vi "DVL convert (SubVI).vi"(0 "String":string) -> (1 "depth":dbl, 3 "dvl alts":dbl[](array[numeric]), 4 "u_wt_dvl":dbl[](array[numeric]), 5 "u_bt_dvl":dbl[](array[numeric]), 6 "SA":dbl[](array[numeric]))   [LabVIEW 2014]
uses:
  Helping Routines/get_set_point (SubVI).vi
panel:
  in  "Reset pressure":bool
  out "BI":dbl[](array[numeric])
  out "WI":dbl[](array[numeric])
  out "RA":dbl[](array[numeric])
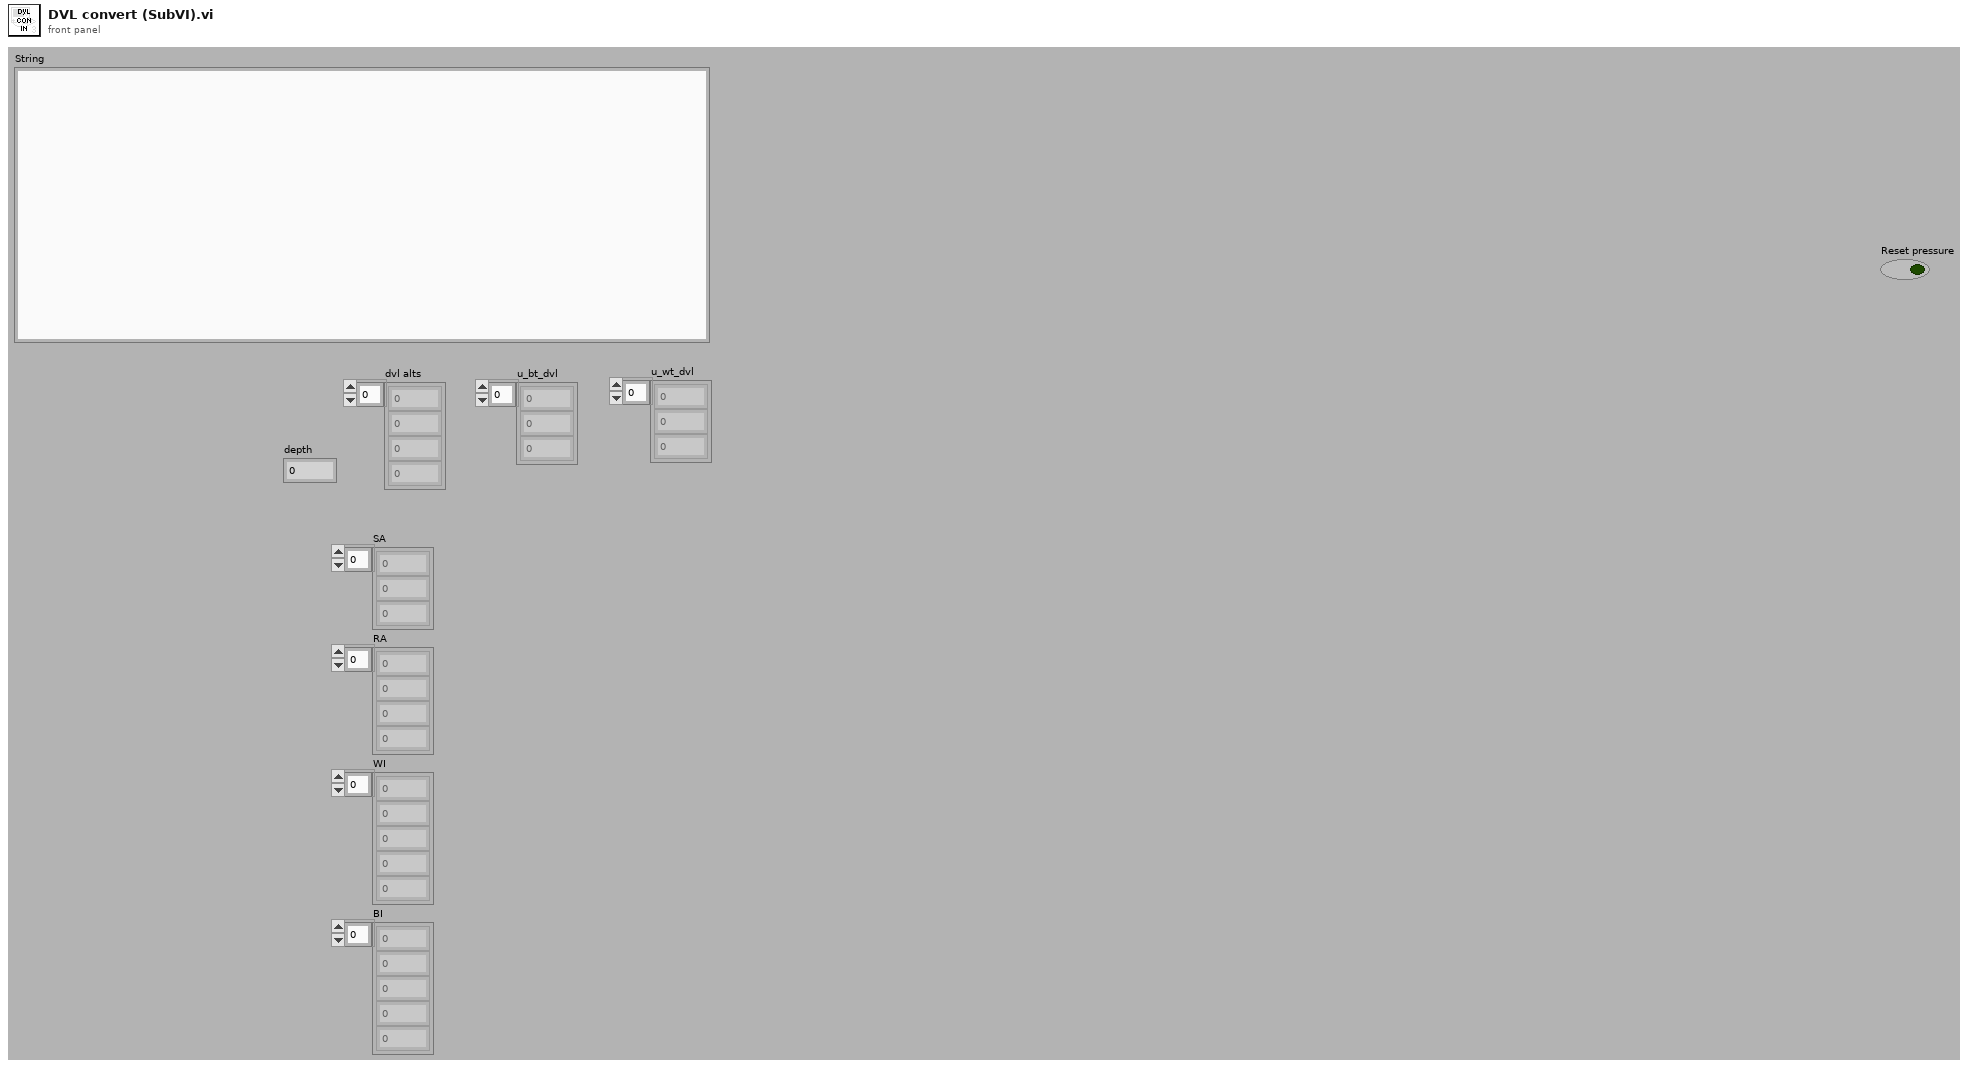
[diagram p1: front panel]
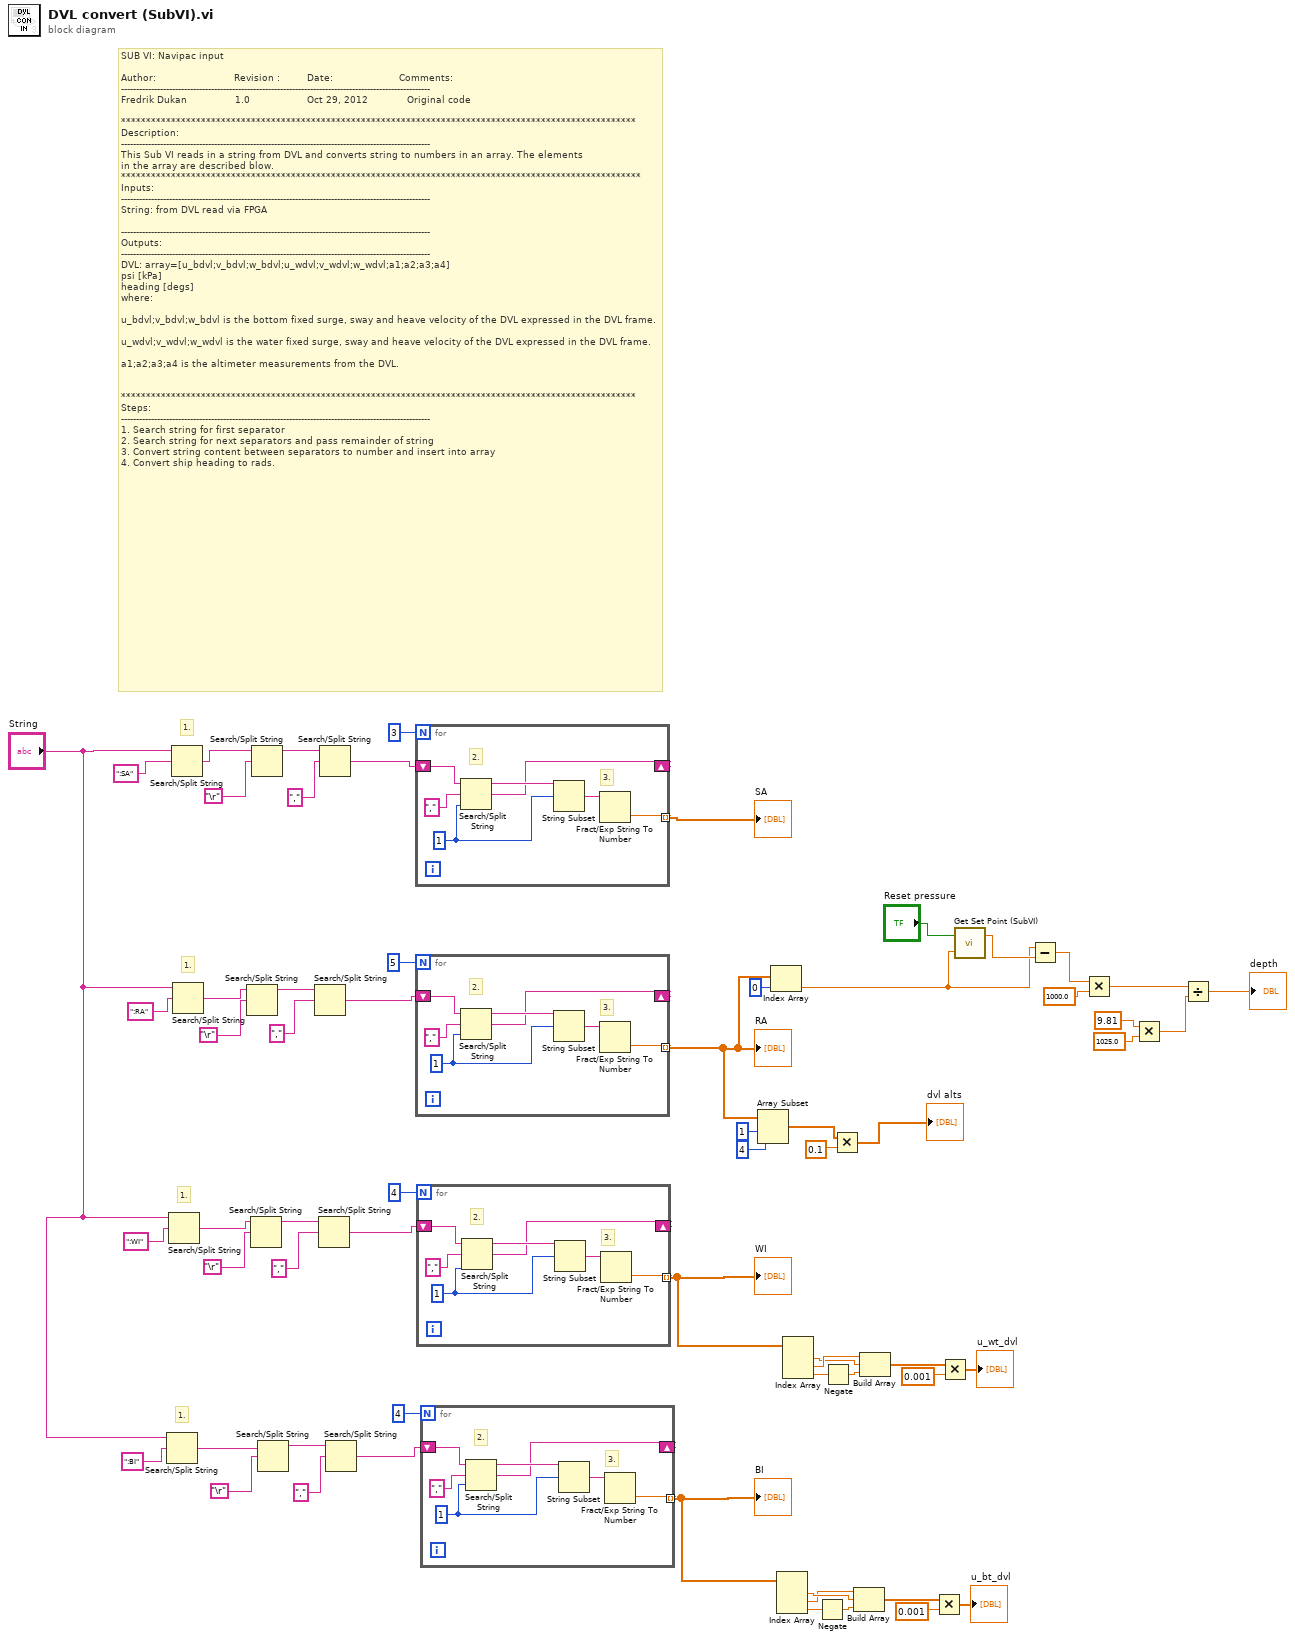
[diagram p0: block diagram]
diagram:
  # "1."
  # "1."
  # "1."
  # "1."
  # "SUB VI: Navipac input\n\nAuthor:                          Revision :         Date:                      Comments:\n-------------------------------------------------------------------------------------------------------\nFredrik Dukan                1.0                   Oct 29, 2012             Original code\n \n*******************************************************************************************************\nDescription:\n-------------------------------------------------------------------------------------------------------\nThis Sub VI reads in a string from DVL and converts string to numbers in an array. The elements\nin the array are described blow.\n********************************************************************************************************\nInputs: \n-------------------------------------------------------------------------------------------------------\nString: from DVL read via FPGA\n\n-------------------------------------------------------------------------------------------------------\nOutputs:  \n-------------------------------------------------------------------------------------------------------\nDVL: array=[u_bdvl;v_bdvl;w_bdvl;u_wdvl;v_wdvl;w_wdvl;a1;a2;a3;a4]\npsi [kPa]\nheading [degs]\nwhere: \n\nu_bdvl;v_bdvl;w_bdvl is the bottom fixed surge, sway and heave velocity of the DVL expressed in the DVL frame.\n\nu_wdvl;v_wdvl;w_wdvl is the water fixed surge, sway and heave velocity of the DVL expressed in the DVL frame.\n\na1;a2;a3;a4 is the altimeter measurements from the DVL.\n\n\n*******************************************************************************************************\nSteps:\n-------------------------------------------------------------------------------------------------------\n1. Search string for first separator \n2. Search string for next separators and pass remainder of string\n3. Convert string content between separators to number and insert into array\n4. Convert ship heading to rads."
  n1 = Search/Split String(string="String", search string/char (-)=":BI") -> (match + rest of string=w12:string)  [unwired: 1 in, 2 out]
  n2 = Search/Split String(string="String", search string/char (-)=":WI") -> (match + rest of string=w16:string)  [unwired: 1 in, 2 out]
  n3 = Search/Split String(string="String", search string/char (-)=":SA") -> (match + rest of string=w58:string)  [unwired: 1 in, 2 out]
  n4 = Search/Split String(string="String", search string/char (-)=":RA") -> (match + rest of string=w20:string)  [unwired: 1 in, 2 out]
  n5 = Search/Split String(string=w20, search string/char (-)="\r") -> (substring before match=w23:string)  [unwired: 1 in, 2 out]
  n6 = Search/Split String(string=w16, search string/char (-)="\r") -> (substring before match=w17:string)  [unwired: 1 in, 2 out]
  n7 = Search/Split String(string=w58, search string/char (-)="\r") -> (substring before match=w24:string)  [unwired: 1 in, 2 out]
  n8 = Search/Split String(string=w12, search string/char (-)="\r") -> (substring before match=w15:string)  [unwired: 1 in, 2 out]
  n9 = Search/Split String(string=w23, search string/char (-)=",") -> (match + rest of string=w10:string)  [unwired: 1 in, 2 out]
  n10 = Search/Split String(string=w17, search string/char (-)=",") -> (match + rest of string=w9:string)  [unwired: 1 in, 2 out]
  n11 = Search/Split String(string=w24, search string/char (-)=",") -> (match + rest of string=w11:string)  [unwired: 1 in, 2 out]
  n12 = Search/Split String(string=w15, search string/char (-)=",") -> (match + rest of string=w8:string)  [unwired: 1 in, 2 out]
  n13 = for {
    N: 3 -> [_]
    shift-right: [w65] -> _
    shift-left: w11 -> [w68]
    tunnel: [w66] -> w52 mode=indexing
    w64 = 1
    # "3."
    # "2."
    n14 = Search/Split String(string=w68, search string/char (-)=",", offset (0)=w64) -> (substring before match=w70:string, match + rest of string=w65:string)  [unwired: 1 out]
    n15 = String Subset(string=w70, offset (0)=w64) -> (substring=w67:string)  [unwired: 1 in]
    n16 = Fract/Exp String To Number(string=w67) -> (number=w66:dbl)  [unwired: 3 in, 1 out]
  }
  "SA" <- w52
  n17 = for {
    N: 5 -> [_]
    shift-right: [w72] -> _
    shift-left: w10 -> [w75]
    tunnel: [w73] -> w33 mode=indexing
    w71 = 1
    # "3."
    # "2."
    n18 = Search/Split String(string=w75, search string/char (-)=",", offset (0)=w71) -> (substring before match=w77:string, match + rest of string=w72:string)  [unwired: 1 out]
    n19 = String Subset(string=w77, offset (0)=w71) -> (substring=w74:string)  [unwired: 1 in]
    n20 = Fract/Exp String To Number(string=w74) -> (number=w73:dbl)  [unwired: 3 in, 1 out]
  }
  "RA" <- w33
  n21 = for {
    N: 4 -> [_]
    shift-right: [w79] -> _
    shift-left: w9 -> [w82]
    tunnel: [w80] -> w42 mode=indexing
    w78 = 1
    # "3."
    # "2."
    n22 = Search/Split String(string=w82, search string/char (-)=",", offset (0)=w78) -> (substring before match=w84:string, match + rest of string=w79:string)  [unwired: 1 out]
    n23 = String Subset(string=w84, offset (0)=w78) -> (substring=w81:string)  [unwired: 1 in]
    n24 = Fract/Exp String To Number(string=w81) -> (number=w80:dbl)  [unwired: 3 in, 1 out]
  }
  "WI" <- w42
  n25 = for {
    N: 4 -> [_]
    shift-right: [w86] -> _
    shift-left: w8 -> [w89]
    tunnel: [w87] -> w51 mode=indexing
    w85 = 1
    # "3."
    # "2."
    n26 = Search/Split String(string=w89, search string/char (-)=",", offset (0)=w85) -> (substring before match=w91:string, match + rest of string=w86:string)  [unwired: 1 out]
    n27 = String Subset(string=w91, offset (0)=w85) -> (substring=w88:string)  [unwired: 1 in]
    n28 = Fract/Exp String To Number(string=w88) -> (number=w87:dbl)  [unwired: 3 in, 1 out]
  }
  "BI" <- w51
  n29 = Array Subset(array=w33, index=1, length=4) -> (w2:dbl[])
  n30 = Index Array(array=w33, index=0) -> (element=w5:dbl)
  n31 = Index Array(array=w51) -> (element #1=w50:dbl, element #2=w49:dbl, element #3=w48:dbl)  [unwired: 3 in]
  n32 = Index Array(array=w42) -> (element #1=w43:dbl, element #2=w44:dbl, element #3=w45:dbl)  [unwired: 3 in]
  n33 = Negate(x=w48) -> (-x=w47:dbl)
  n34 = Negate(x=w45) -> (-x=w46:dbl)
  n35 = Multiply(x=w2, y=0.1) -> (x*y=→"dvl alts":dbl[])
  n36 = Build Array(w49, w50, w47) -> (w35:dbl[])
  n37 = Build Array(w44, w43, w46) -> (w38:dbl[])
  n38 = Multiply(x=w35, y=0.001) -> (x*y=→"u_bt_dvl":dbl[])
  n39 = Multiply(x=w38, y=0.001) -> (x*y=→"u_wt_dvl":dbl[])
  n40 = call-poly "Get Set Point (SubVI).vi"("set point in"=w5, "auto set  in"="Reset pressure") -> ("set point"=w6:dbl)  [unwired: 1 out]
  n41 = Subtract(x=w5, y=w6) -> (x-y=w4:dbl)
  n42 = Multiply(x=w4, y=1000.0) -> (x*y=w28:dbl)
  n43 = Multiply(x=9.81, y=1025.0) -> (x*y=w27:dbl)
  n44 = Divide(x=w28, y=w27) -> (x/y=→"depth":dbl)
